vi "core.vi"(8 "ABCD in":u32[](array[numeric]) format="%.0x", 11 "M[ ]":u32[](array[numeric]) format="%.0x") -> (0 "ABCD out":u32[](array[numeric]) format="%.0x")   [LabVIEW 2013, in "MD5.lvlib" / "MD5.lvclass"]
uses:
  MD5.lvclass
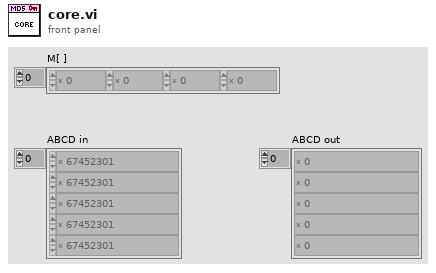
[diagram p1: front panel]
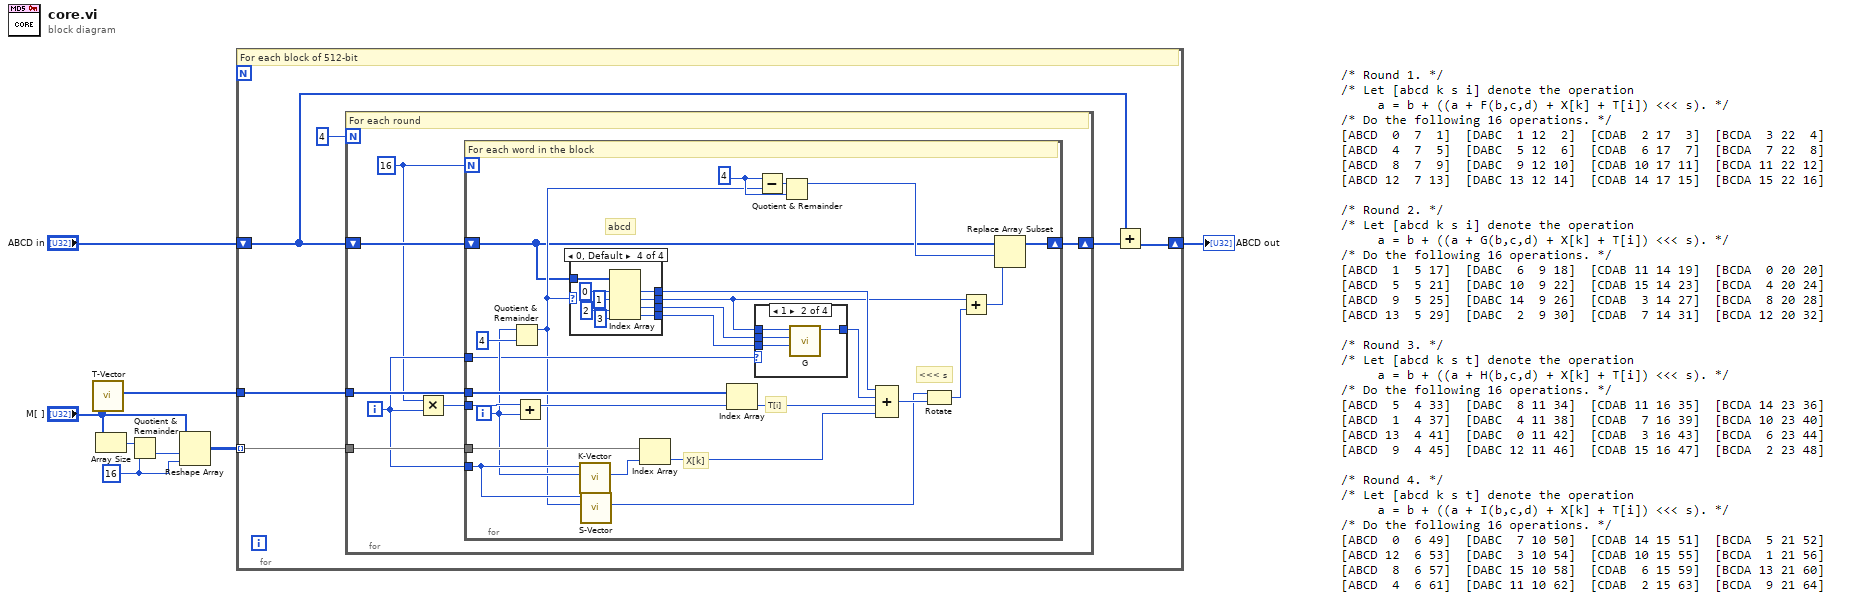
[diagram p0: block diagram]
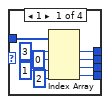
[diagram p2: hidden frame]
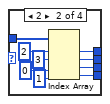
[diagram p3: hidden frame]
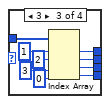
[diagram p4: hidden frame]
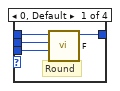
[diagram p5: hidden frame]
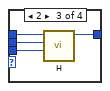
[diagram p6: hidden frame]
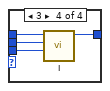
[diagram p7: hidden frame]
diagram:
  w2 = 16 ("y")
  n1 = call "T-Vector.vi"() -> ("T"=w5:u32[])  [unwired: 11 in]
  n2 = Array Size(array="M[ ]") -> (size(s)=w6:i32)
  n3 = Quotient & Remainder(x=w6, y=w2) -> (floor(x/y)=w4:i32)  [unwired: 1 out]
  n4 = Reshape Array("M[ ]", w4, w2) -> (w3:u32[][])
  n5 = for {
    shift-right: [w13] -> w7
    shift-left: "ABCD in" -> [w14]
    tunnel: w5 -> [w10]
    tunnel: w3 -> [w9] mode=indexing
    # "For each block of 512-bit"
    n6 = for {
      N: 4 -> [_]
      shift-right: [w16] -> w12
      shift-left: w14 -> [w21]
      tunnel: w9 -> [w18]
      tunnel: w10 -> [w20]
      i -> [w17]
      w15 = 16
      # "For each round"
      n7 = Multiply(x=w15, y=w17) -> (x*y=w19:i32)
      n8 = for {
        N: w15 -> [_]
        shift-right: [w29] -> w16
        shift-left: w21 -> [w26]
        tunnel: w20 -> [w47]
        tunnel: w19 -> [w46]
        tunnel: w17 -> [w41]
        tunnel: w18 -> [w45]
        tunnel: w17 -> [w35]
        i -> [w39]
        w38 = 4 ("y")
        # "<<< s"
        # "abcd"
        # "X[k]"
        # "T[i]"
        # "For each word in the block"
        n9 = Quotient & Remainder(x=w39, y=4) -> (x-y*floor(x/y)=w27:i32)  [unwired: 1 out]
        n10 = Add(x=w46, y=w39) -> (x+y=w40:i32)
        n11 = case shown="0, Default" w27 {
          tunnel: w26 -> [w56 w65 w74 w83]
          tunnel: [w55 w64 w73 w82] -> w25
          tunnel: [w54 w63 w72 w81] -> w24
          tunnel: [w53 w62 w71 w80] -> w23
          tunnel: [w52 w61 w70 w79] -> w22
          frame 1 {
            n12 = Index Array(array=w56, index #1=3 ("index"), index #2=0 ("index"), index #3=1 ("index"), index #4=2 ("index")) -> (element #1=w55:u32, element #2=w54:u32, element #3=w53:u32, element #4=w52:u32)
          }
          frame 2 {
            n13 = Index Array(array=w65, index #1=2 ("index"), index #2=3 ("index"), index #3=0 ("index"), index #4=1 ("index")) -> (element #1=w64:u32, element #2=w63:u32, element #3=w62:u32, element #4=w61:u32)
          }
          frame 3 {
            n14 = Index Array(array=w74, index #1=1 ("index"), index #2=2 ("index"), index #3=3 ("index"), index #4=0 ("index")) -> (element #1=w73:u32, element #2=w72:u32, element #3=w71:u32, element #4=w70:u32)
          }
          frame 0, Default {
            n15 = Index Array(array=w83, index #1=0 ("index"), index #2=1 ("index"), index #3=2 ("index"), index #4=3 ("index")) -> (element #1=w82:u32, element #2=w81:u32, element #3=w80:u32, element #4=w79:u32)
          }
        }
        n16 = call "K-Vector.vi"("i-th word"=w39, "Round"=w41) -> ("k"=w44:i32)  [unwired: 9 in]
        n17 = call "S-Vector.vi"("i-th word"=w27, "Round"=w41) -> ("s"=w31:i32)  [unwired: 9 in]
        n18 = Index Array(array=w45, index=w44) -> (element=w28:u32)
        n19 = Index Array(array=w47, index=w40) -> (element=w32:u32)
        n20 = case shown="1" w35 {
          tunnel: [w87 w88 w92 w98] -> w33
          tunnel: w22 -> [w86 w89 w93 w96]
          tunnel: w23 -> [w85 w90 w94 w97]
          tunnel: w24 -> [w84 w91 w95 w99]
          frame 0, Default {
            # "Round"
            n21 = call "F.vi"("Z"=w86, "Y"=w85, "X"=w84) -> ("F"=w87:u32)  [unwired: 8 in]
          }
          frame 1 {
            n22 = call "G.vi"("Z"=w89, "Y"=w90, "X"=w91) -> ("G"=w88:u32)  [unwired: 8 in]
          }
          frame 2 {
            n23 = call "H.vi"("Z"=w93, "Y"=w94, "X"=w95) -> ("H"=w92:u32)  [unwired: 8 in]
          }
          frame 3 {
            n24 = call "I.vi"("Z"=w96, "Y"=w97, "X"=w99) -> ("I"=w98:u32)  [unwired: 8 in]
          }
        }
        n25 = Subtract(x=w38, y=w27) -> (x-y=w37:i32)
        n26 = Quotient & Remainder(x=w37, y=w38) -> (x-y*floor(x/y)=w36:i32)  [unwired: 1 out]
        n27 = Compound Arithmetic op=ADD(w25, w33, w32, w28) -> (w34:u32)
        n28 = Rotate(1:w34, 2:w31) -> (0:w30:u32)
        n29 = Add(x=w24, y=w30) -> (x+y=w43:u32)
        n30 = Replace Array Subset(array=w26, new element=w43, index=w36) -> (w29:u32[])
      }
    }
    n31 = Add(x=w14, y=w12) -> (x+y=w13:u32[])
  }
  "ABCD out" <- w7
